vi "Linear interpolation.vi"(2 "Yf":i32=15, 3 "Y0":i32, 4 "Xf":i32=10, 5 "X0":i32) -> (0 "Y array":i32[](array[numeric])=[0, 0, 1, 2, 2, 3, 3, 4, 5, 5, 6, 6, 7, 8, 8, 9, 9, 10, 11, 11, 12, 12, 13, 14, 14, 15], 1 "X array":i32[](array[numeric])=[0, 1, 1, 1, 2, 2, 3, 3, 3, 4, 4, 5, 5, 5, 6, 6, 7, 7, 7, 8, 8, 9, 9, 9, 10, 10])   [LabVIEW 2019]
panel:
  out "XY Graph":cluster{i32[], i32[]}(graph)={[0, 1, 1, 1, 2, 2, 3, 3, 3, 4, 4, 5, 5, 5, 6, 6, 7, 7, 7, 8, 8, 9, 9, 9, 10, 10], [0, 0, 1, 2, 2, 3, 3, 4, 5, 5, 6, 6, 7, 8, 8, 9, 9, 10, 11, 11, 12, 12, 13, 14, 14, 15]}
  # "Начальная точка"
  # "Конечная точка"
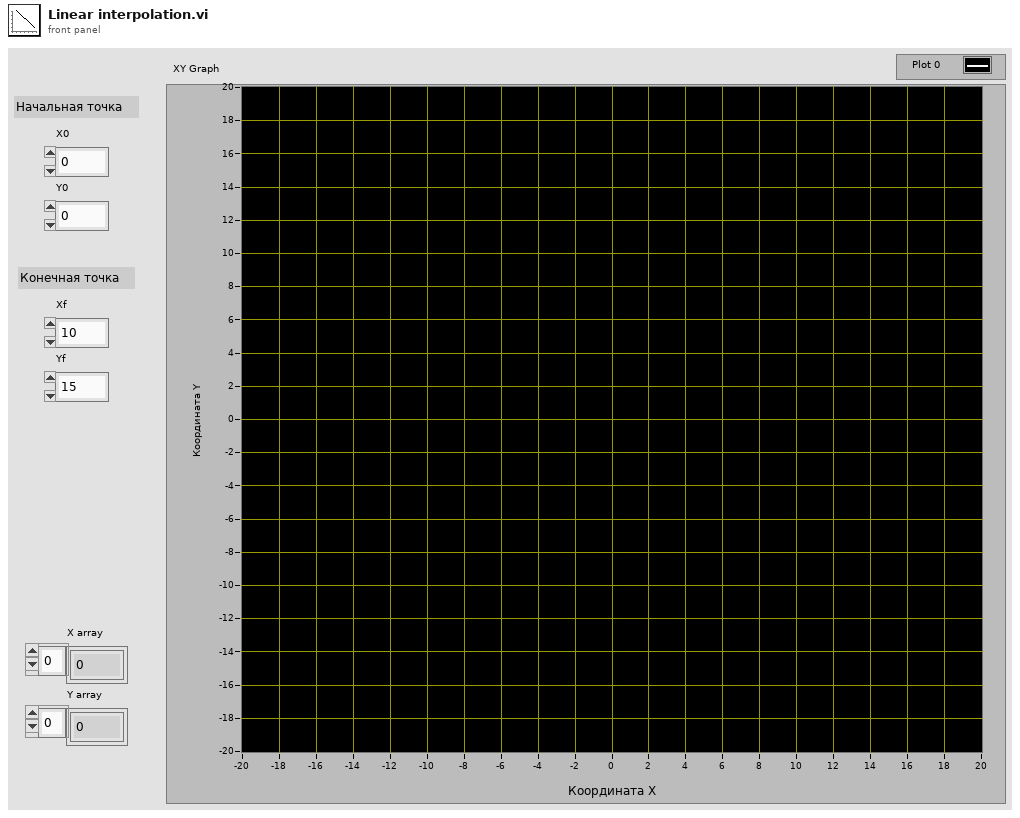
[diagram p1: front panel]
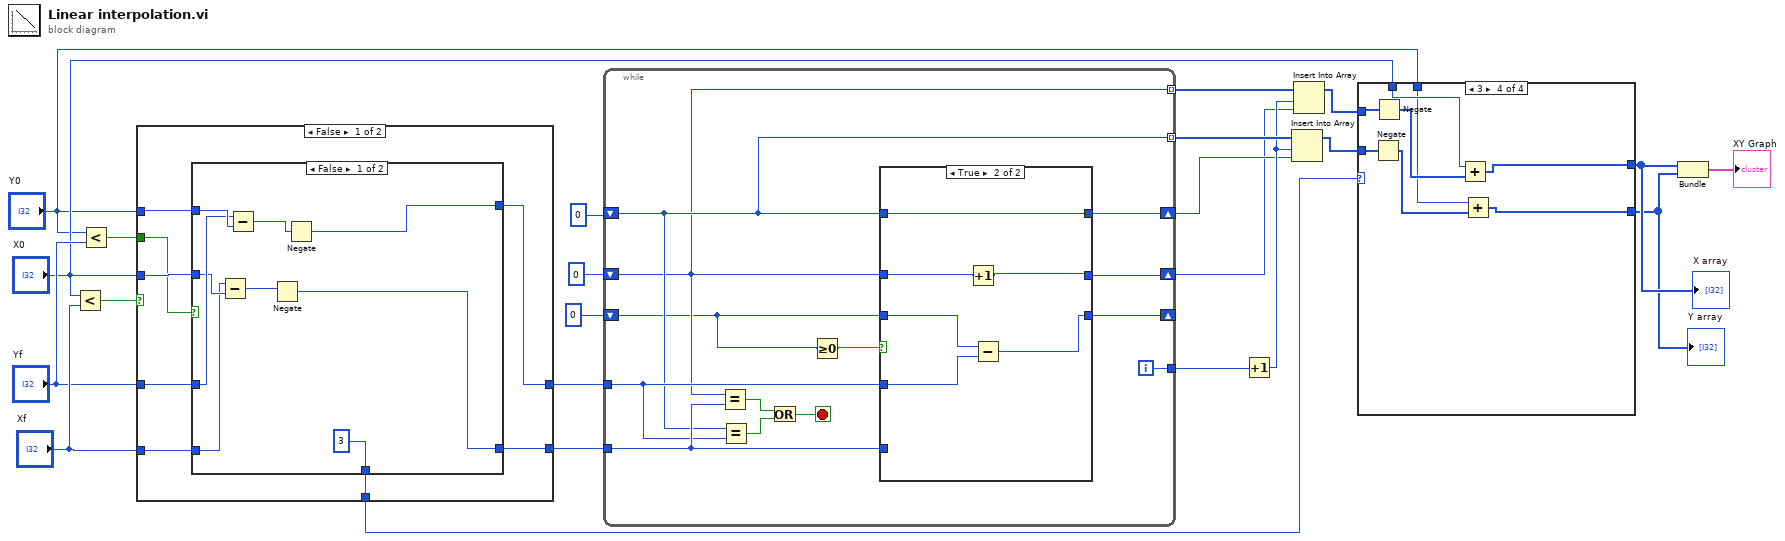
[diagram p0: block diagram]
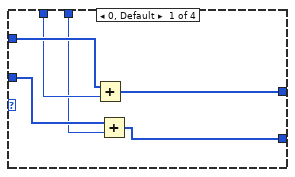
[diagram p2: hidden frame]
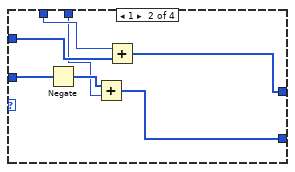
[diagram p3: hidden frame]
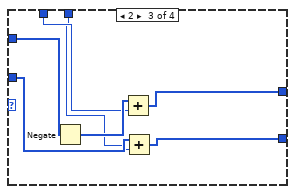
[diagram p4: hidden frame]
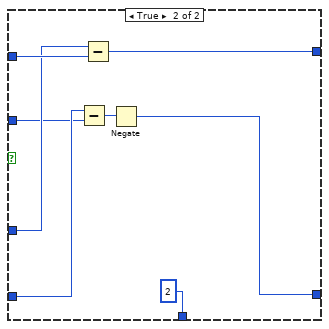
[diagram p5: hidden frame]
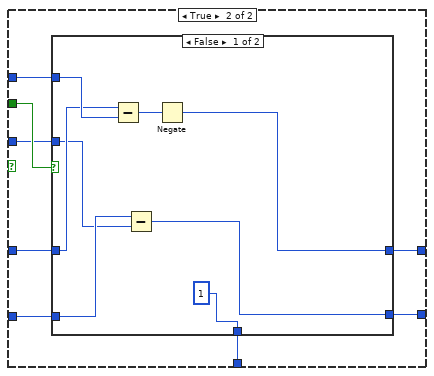
[diagram p6: hidden frame]
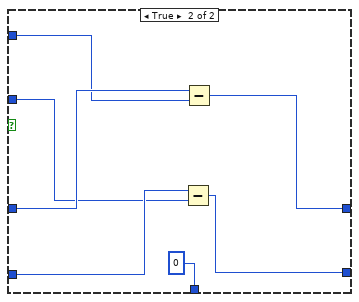
[diagram p7: hidden frame]
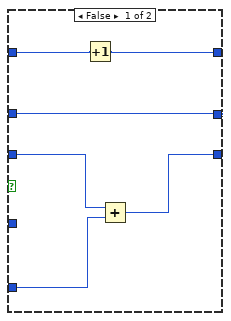
[diagram p8: hidden frame]
diagram:
  n1 = Less?(x="X0", y="Xf") -> (x < y?=w14:bool)
  n2 = Less?(x="Y0", y="Yf") -> (x < y?=w13:bool)
  n3 = case shown="False" w14 {
    tunnel: w13 -> [w27 w56]
    tunnel: "Xf" -> [w29 w52]
    tunnel: "Yf" -> [w30 w53]
    tunnel: "X0" -> [w28 w54]
    tunnel: "Y0" -> [w31 w55]
    tunnel: [w25 w51] -> w10
    tunnel: [w26 w50] -> w9
    tunnel: [w24 w49] -> w8
    frame False {
      n4 = case shown="False" w27 {
        tunnel: w31 -> [w40 w48]
        tunnel: w30 -> [w39 w47]
        tunnel: w29 -> [w37 w46]
        tunnel: w28 -> [w38 w45]
        tunnel: [w34 w43] -> w26
        tunnel: [w33 w42] -> w25
        tunnel: [3 2] -> w24
        frame False {
          n5 = Subtract(x=w37, y=w38) -> (x-y=w35:i32)
          n6 = Subtract(x=w39, y=w40) -> (x-y=w36:i32)
          n7 = Negate(x=w35) -> (-x=w34:i32)
          n8 = Negate(x=w36) -> (-x=w33:i32)
        }
        frame True {
          n9 = Subtract(x=w46, y=w45) -> (x-y=w44:i32)
          n10 = Subtract(x=w47, y=w48) -> (x-y=w42:i32)
          n11 = Negate(x=w44) -> (-x=w43:i32)
        }
      }
    }
    frame True {
      n12 = case shown="False" w56 {
        tunnel: w55 -> [w64 w70]
        tunnel: w54 -> [w61 w68]
        tunnel: w53 -> [w63 w71]
        tunnel: w52 -> [w62 w69]
        tunnel: [w59 w67] -> w51
        tunnel: [w58 w66] -> w50
        tunnel: [1 0] -> w49
        frame False {
          n13 = Subtract(x=w63, y=w64) -> (x-y=w60:i32)
          n14 = Subtract(x=w62, y=w61) -> (x-y=w58:i32)
          n15 = Negate(x=w60) -> (-x=w59:i32)
        }
        frame True {
          n16 = Subtract(x=w69, y=w68) -> (x-y=w66:i32)
          n17 = Subtract(x=w71, y=w70) -> (x-y=w67:i32)
        }
      }
    }
  }
  n18 = while {
    shift-right: [w80] -> w18
    shift-left: 0 -> [w75]
    shift-right: [w81] -> w17
    shift-left: 0 -> [w74]
    shift-right: [w79] -> _
    shift-left: 0 -> [w72]
    tunnel: w9 -> [w78]
    tunnel: w10 -> [w77]
    tunnel: [w76] -> w22
    tunnel: [w74] -> w21 mode=indexing
    tunnel: [w75] -> w20 mode=indexing
    i -> [w76]
    stop <- w84 stop-if-true
    n19 = Equal?(x=w74, y=w78) -> (x = y?=w83:bool)
    n20 = Equal?(x=w75, y=w77) -> (x = y?=w82:bool)
    n21 = Or(x=w83, y=w82) -> (x .or. y?=w84:bool)
    n22 = Greater Or Equal To 0?(x=w72) -> (x >= 0?=w73:bool)
    n23 = case shown="True" w73 {
      tunnel: w72 -> [w90 w92]
      tunnel: w75 -> [w85 w96]
      tunnel: [w89 w95] -> w81
      tunnel: w74 -> [w89 w94]
      tunnel: [w86 w96] -> w80
      tunnel: [w88 w93] -> w79
      tunnel: w78 -> [w87 _]
      tunnel: w77 -> [_ w91]
      frame False {
        n24 = Increment(x=w85) -> (x+1=w86:i32)
        n25 = Add(x=w90, y=w87) -> (x+y=w88:i32)
      }
      frame True {
        n26 = Increment(x=w94) -> (x+1=w95:i32)
        n27 = Subtract(x=w92, y=w91) -> (x-y=w93:i32)
      }
    }
  }
  n28 = Increment(x=w22) -> (x+1=w19:i32)
  n29 = Insert Into Array(array=w20, index=w19, new element=w18) -> (w6:i32[])
  n30 = Insert Into Array(array=w21, index=w19, new element=w17) -> (w7:i32[])
  n31 = case shown="3" w8 {
    tunnel: w7 -> [w102 w108 w116 w123]
    tunnel: w6 -> [w101 w109 w113 w124]
    tunnel: "X0" -> [w100 w107 w114 w122]
    tunnel: "Y0" -> [w99 w105 w112 w120]
    tunnel: [w98 w104 w111 w118] -> w2
    tunnel: [w97 w103 w110 w117] -> w1
    frame 0, Default {
      n32 = Add(x=w102, y=w100) -> (x+y=w98:i32[])
      n33 = Add(x=w101, y=w99) -> (x+y=w97:i32[])
    }
    frame 1 {
      n34 = Negate(x=w109) -> (-x=w106:i32[])
      n35 = Add(x=w106, y=w105) -> (x+y=w103:i32[])
      n36 = Add(x=w107, y=w108) -> (x+y=w104:i32[])
    }
    frame 2 {
      n37 = Negate(x=w116) -> (-x=w115:i32[])
      n38 = Add(x=w115, y=w114) -> (x+y=w111:i32[])
      n39 = Add(x=w113, y=w112) -> (x+y=w110:i32[])
    }
    frame 3 {
      n40 = Negate(x=w124) -> (-x=w119:i32[])
      n41 = Negate(x=w123) -> (-x=w121:i32[])
      n42 = Add(x=w122, y=w121) -> (x+y=w118:i32[])
      n43 = Add(x=w120, y=w119) -> (x+y=w117:i32[])
    }
  }
  "X array" <- w2
  "Y array" <- w1
  n44 = Bundle(w2, w1) -> (→"XY Graph":cluster{i32[], i32[]})  [unwired: 1 in]
